vi "Update Run Service.vi"(8 "error in (no error)":errorcluster, 10 "User Service Library in":refnum<vi>, 11 "Generated Server Library in":refnum<vi>) -> (0 "error out":errorcluster)   [LabVIEW 2019, in "gRPC Template Creation Utility.lvlib"]
uses:
  gRPC Template Creation Utility.lvlib
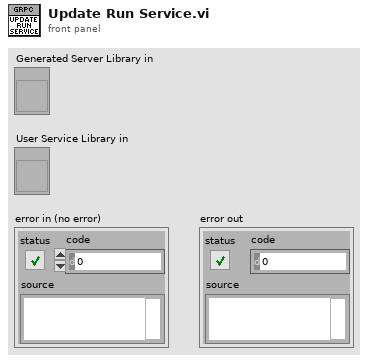
[diagram p1: front panel]
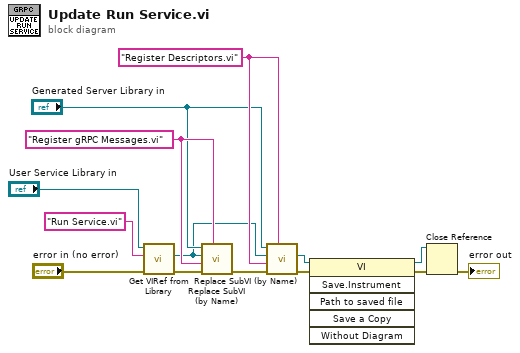
[diagram p0: block diagram]
diagram:
  w7 = "Register Descriptors.vi"
  w8 = "Register gRPC Messages.vi"
  n1 = call "Get VIRef from Library.vi"("error in (no error)"="error in (no error)", "Item Name"="Run Service.vi", "Library"="User Service Library in") -> ("error out"=w12:errorcluster, "VIref out"=w5:refnum<vi>)  [unwired: 5 in, 2 out]
  n2 = call "Replace SubVI (by Name).vi"("SubVI to replace with"=w8, "error in (no error)"=w12, "SubVI being replaced"=w8, "VI in"=w5, "Library in"="Generated Server Library in") -> ("error out"=w4:errorcluster)  [unwired: 4 in, 2 out]
  n3 = call "Replace SubVI (by Name).vi"("SubVI to replace with"=w7, "error in (no error)"=w4, "SubVI being replaced"=w7, "VI in"=w5, "Library in"="Generated Server Library in") -> ("error out"=w3:errorcluster, "VI out"=w2:refnum<vi>)  [unwired: 4 in, 1 out]
  n4 = invoke class="VI" method="Save.Instrument"(reference=w2, error in=w3) -> (reference out=w1:refnum<vi>, error out=w14:errorcluster)  [unwired: 4 in, 4 out]
  n5 = Close Reference(reference=w1, error in (no error)=w14) -> (error out=→"error out":errorcluster)
